vi "raw2Json.vi"(8 "error in":errorcluster, 10 "rawData":string[][](array[string]), 11 "TGA/DSC":T1) -> (0 "error in 2":errorcluster caption="error out", 3 "fullJson":string)   [LabVIEW 2011]
uses:
  dataType/TGA_DSC.ctl
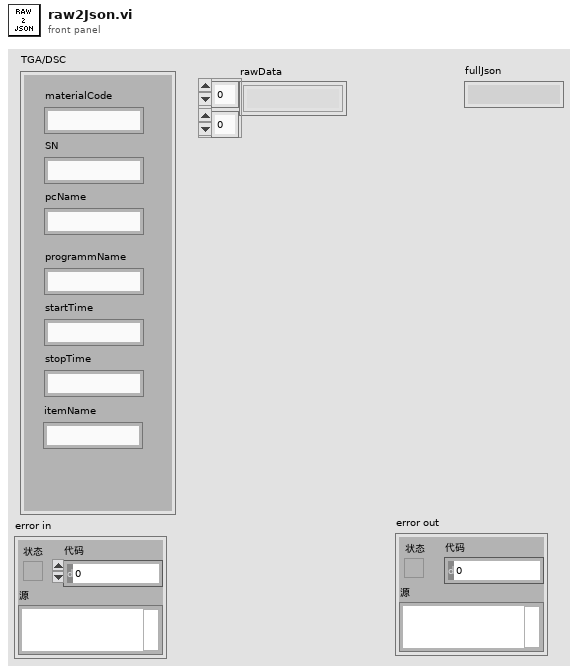
[diagram p1: front panel]
types:
  T1 = typedef "TGA_DSC.ctl" = cluster{"materialCode":string, "SN":string, "pcName":string, "programmName":string, "startTime":string, "stopTime":string, "itemName":string}
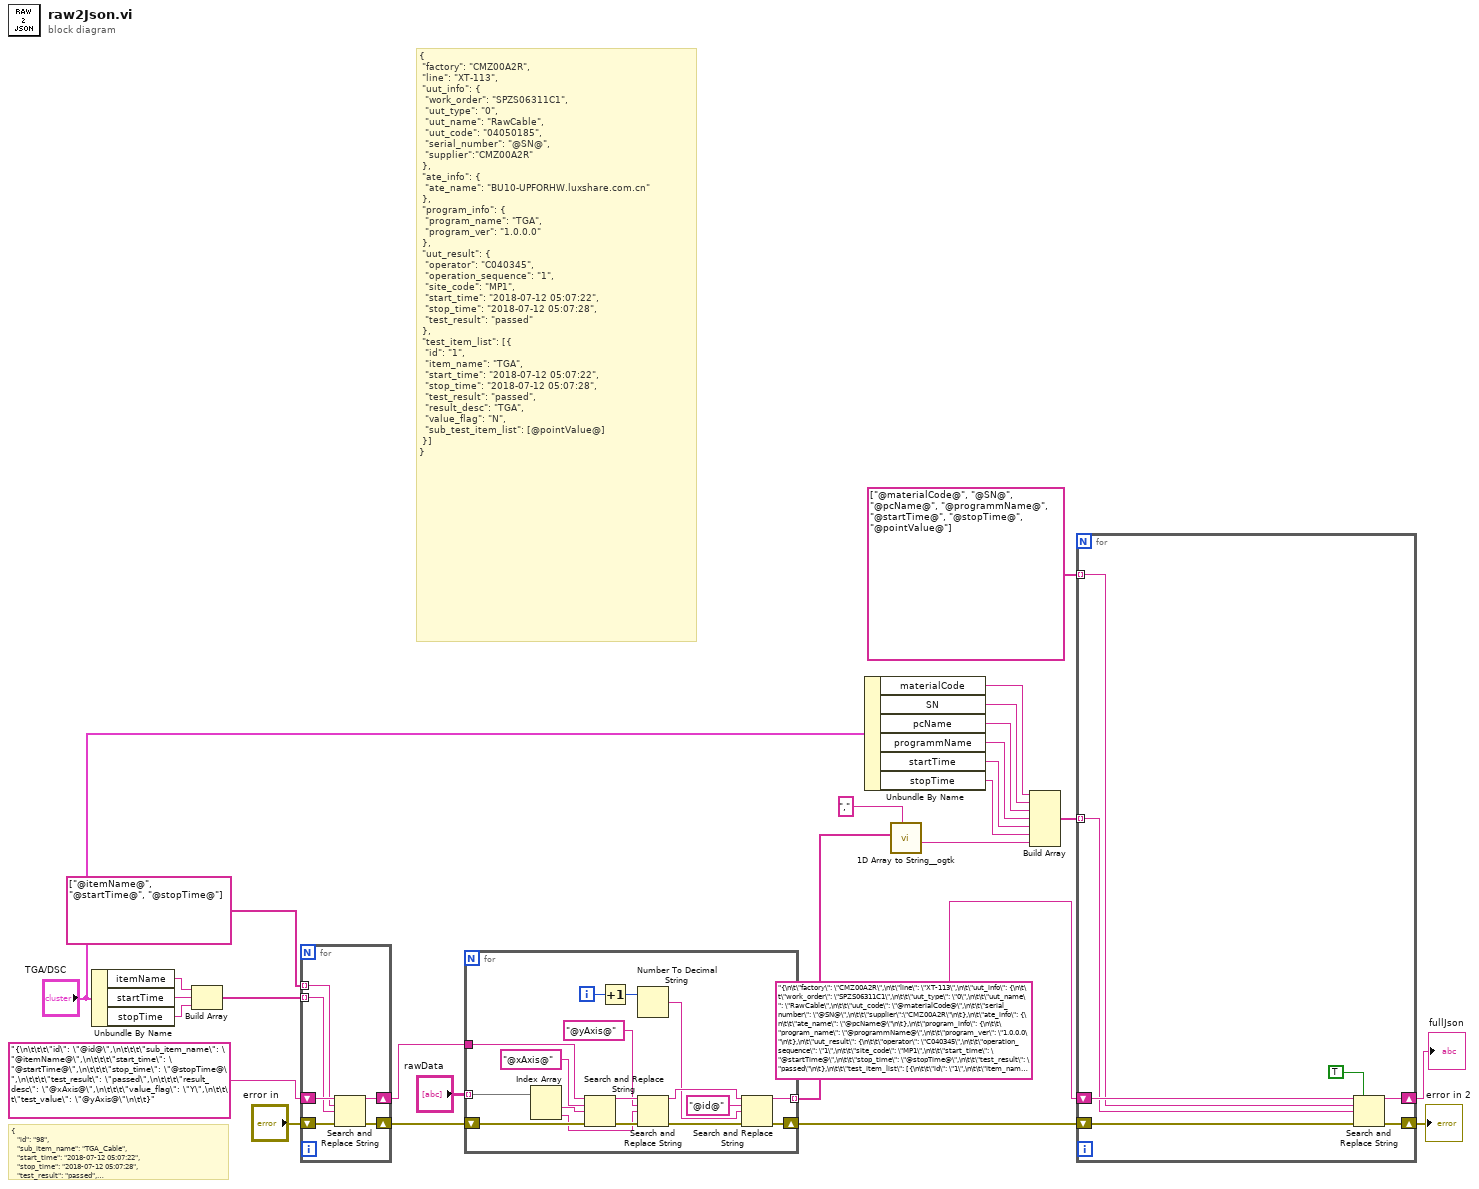
[diagram p0: block diagram]
diagram:
  # "{\n\t\"factory\": \"CMZ00A2R\",\n\t\"line\": \"XT-113\",\n\t\"uut_info\": {\n\t\t\"work_order\": \"SPZS06311C1\",\n\t\t\"uut_type\": \"0\",\n\t\t\"uut_name\": \"RawCable\",\n\t\t\"uut_code\": \"04050185\",\n\t\t\"serial_number\": \"@SN@\",\n\t\t\"supplier\":\"CMZ00A2R\"\n\t},\n\t\"ate_info\": {\n\t\t\"ate_name\": \"BU10-UPFORHW.luxshare.com.cn\"\n\t},\n\t\"program_info\": {\n\t\t\"program_name\": \"TGA\",\n\t\t\"program_ver\": \"1.0.0.0\"\n\t},\n\t\"uut_result\": {\n\t\t\"operator\": \"C040345\",\n\t\t\"operation_sequence\": \"1\",\n\t\t\"site_code\": \"MP1\",\n\t\t\"start_time\": \"2018-07-12 05:07:22\",\n\t\t\"stop_time\": \"2018-07-12 05:07:28\",\n\t\t\"test_result\": \"passed\"\n\t},\n\t\"test_item_list\": [{\n\t\t\"id\": \"1\",\n\t\t\"item_name\": \"TGA\",\n\t\t\"start_time\": \"2018-07-12 05:07:22\",\n\t\t\"stop_time\": \"2018-07-12 05:07:28\",\n\t\t\"test_result\": \"passed\",\n\t\t\"result_desc\": \"TGA\",\n\t\t\"value_flag\": \"N\",\n\t\t\"sub_test_item_list\": [@pointValue@]\n\t}]\n}"
  # "{\n\t\t\t\"id\": \"98\",\n\t\t\t\"sub_item_name\": \"TGA_Cable\",\n\t\t\t\"start_time\": \"2018-07-12 05:07:22\",\n\t\t\t\"stop_time\": \"2018-07-12 05:07:28\",\n\t\t\t\"test_result\": \"passed\",\n\t\t\t\"result_desc\": \"838.333\",\n\t\t\t\"value_flag\": \"Y\",\n\t\t\t\"test_value\": \"2.2434\"\n\t\t}"
  n1 = Unbundle By Name("TGA/DSC") -> ("itemName"=w17:string, "startTime"=w16:string, "stopTime"=w15:string)
  n2 = Build Array(w17, w16, w15) -> (w24:string[])
  n3 = for {
    tunnel: string[] ["@itemName@", "@startTime@", "@stopTime@"] -> [w31] mode=indexing
    tunnel: w24 -> [w30] mode=indexing
    shift-right: [w29] -> w22
    shift-left: "{\n\t\t\t\"id\": \"@id@\",\n\t\t\t\"sub_item_name\": \"@itemName@\",\n\t\t\t\"start_time\": \"@startTime@\",\n\t\t\t\"stop_time\": \"@stopTime@\",\n\t\t\t\"test_result\": \"passed\",\n\t\t\t\"result_desc\": \"@xAxis@\",\n\t\t\t\"value_flag\": \"Y\",\n\t\t\t\"test_value\": \"@yAxis@\"\n\t\t}" -> [w32]
    shift-right: [w28] -> w21
    shift-left: "error in" -> [w27]
    n4 = Search and Replace String(input string=w32, search string=w31, replace string=w30, error in=w27) -> (result string=w29:string, error out=w28:errorcluster)  [unwired: 4 in, 2 out]
  }
  n5 = for {
    tunnel: "rawData" -> [w45] mode=indexing
    tunnel: w22 -> [w47]
    shift-right: [w33] -> w5
    shift-left: w21 -> [w43]
    tunnel: [w34] -> w20 mode=indexing
    i -> [w49]
    n6 = Index Array(array=w45) -> (element #1=w44:string, element #2=w39:string)  [unwired: 2 in]
    n7 = Search and Replace String(input string=w47, search string="@xAxis@" ("搜索字符串"), replace string=w44, error in=w43) -> (result string=w42:string, error out=w41:errorcluster)  [unwired: 4 in, 2 out]
    n8 = Increment(x=w49) -> (x+1=w48:i32)
    n9 = Number To Decimal String(number=w48) -> (decimal integer string=w36:string)  [unwired: 1 in]
    n10 = Search and Replace String(input string=w42, search string="@yAxis@" ("搜索字符串"), replace string=w39, error in=w41) -> (result string=w38:string, error out=w35:errorcluster)  [unwired: 4 in, 2 out]
    n11 = Search and Replace String(input string=w38, search string="@id@" ("搜索字符串"), replace string=w36, error in=w35) -> (result string=w34:string, error out=w33:errorcluster)  [unwired: 4 in, 2 out]
  }
  n12 = Unbundle By Name("TGA/DSC") -> ("materialCode"=w13:string, "SN"=w12:string, "pcName"=w11:string, "programmName"=w10:string, "startTime"=w9:string, "stopTime"=w8:string)
  n13 = call <userlib>:"1D Array to String__ogtk.vi"("delimiter (Tab)"=",", "Array of Strings"=w20) -> ("delimited string"=w7:string)  [unwired: 9 in]
  n14 = Build Array(w13, w12, w11, w10, w9, w8, w7) -> (w6:string[])
  n15 = for {
    tunnel: string[] ["@materialCode@", "@SN@", "@pcName@", "@programmName@", "@startTime@", "@stopTime@", "@pointValue@"] -> [w54] mode=indexing
    shift-right: [w55] -> w3
    shift-left: "{\n\t\"factory\": \"CMZ00A2R\",\n\t\"line\": \"XT-113\",\n\t\"uut_info\": {\n\t\t\"work_order\": \"SPZS06311C1\",\n\t\t\"uut_type\": \"0\",\n\t\t\"uut_name\": \"RawCable\",\n\t\t\"uut_code\": \"@materialCode@\",\n\t\t\"serial_number\": \"@SN@\",\n\t\t\"supplier\":\"CMZ00A2R\"\n\t},\n\t\"ate_info\": {\n\t\t\"ate_name\": \"@pcName@\"\n\t},\n\t\"program_info\": {\n\t\t\"program_name\": \"@programmName@\",\n\t\t\"program_ver\": \"1.0.0.0\"\n\t},\n\t\"uut_result\": {\n\t\t\"operator\": \"C040345\",\n\t\t\"operation_sequence\": \"1\",\n\t\t\"site_code\": \"MP1\",\n\t\t\"start_time\": \"@startTime@\",\n\t\t\"stop_time\": \"@stopTime@\",\n\t\t\"test_result\": \"passed\"\n\t},\n\t\t\"test_item_list\": [{\n\t\t\"id\": \"1\",\n\t\t\"item_name\": \"@programmName@\",\n\t\t\"start_time\": \"@startTime@\",\n\t\t\"stop_time\": \"@stopTime@\",\n\t\t\"test_result\": \"passed\",\n\t\t\"result_desc\": \"@programmName@\",\n\t\t\"value_flag\": \"N\",\n\t\t\"sub_test_item_list\": [@pointValue@]\n\t}]\n}" -> [w56]
    tunnel: w6 -> [w53] mode=indexing
    shift-right: [w51] -> w1
    shift-left: w5 -> [w52]
    n16 = Search and Replace String(replace all?=TRUE ("替换全部？(F)"), input string=w56, search string=w54, replace string=w53, error in=w52) -> (result string=w55:string, error out=w51:errorcluster)  [unwired: 3 in, 2 out]
  }
  "fullJson" <- w3
  "error in 2" <- w1
